vi "NodosPropiedad_Graficas.vi"() -> ()   [LabVIEW 2020]
uses:
  <vilib>/numeric/Random Number (Range) I64.vi
  <vilib>/numeric/sub_Random U32.vi
panel:
  out "Date and Time":string
  in  "Abort":bool
  in  "limite alto":dbl
  in  "Sample Rate (ms)":u32
  in  "Points to Acquired":i32
  out "Point Acquired":i32
  out "Fuera de rango":bool
  out "Temperatura":cluster{"number":i64, "limite alto":dbl}(graph)
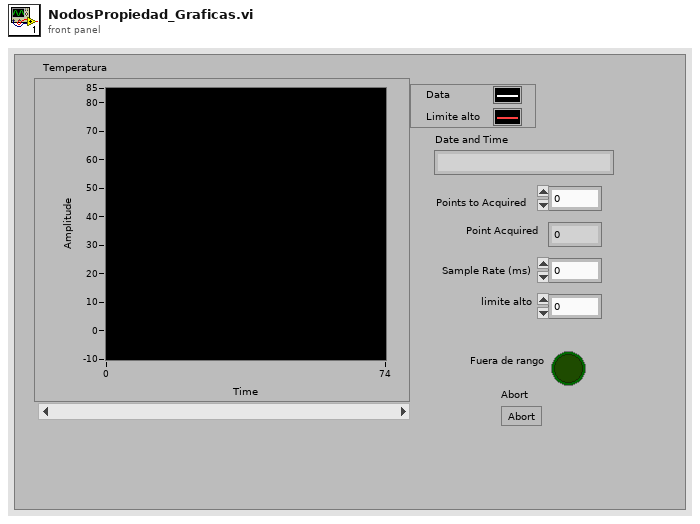
[diagram p1: front panel]
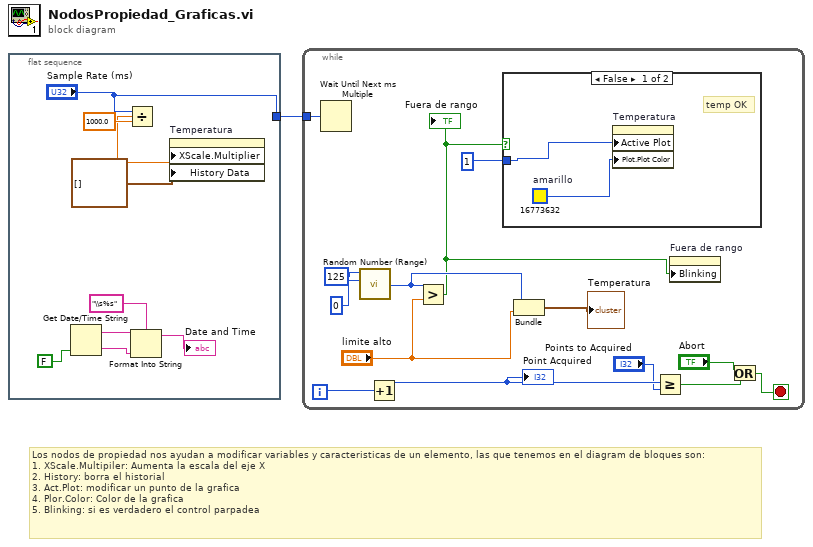
[diagram p0: block diagram]
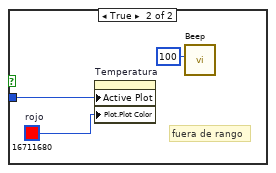
[diagram p2: hidden frame]
diagram:
  # "Los nodos de propiedad nos ayudan a modificar variables y caracteristicas de un elemento, las que tenemos en el diagram de bloques son:\n1. XScale.Multipiler: Aumenta la escala del eje X\n2. History: borra el historial  \n3. Act.Plot: modificar un punto de la grafica \n4. Plor.Color: Color de la grafica \n5. Blinking: si es verdadero el control parpadea"
  n1 = flat-sequence {
    tunnel: ["Sample Rate (ms)"] -> w1
    frame #0 {
      n2 = Get Date/Time String(want seconds? (F)=FALSE) -> (date string=w5:string, time string=w4:string)  [unwired: 2 in]
      n3 = Divide(x="Sample Rate (ms)", y=1000.0) -> (x/y=w9:dbl)
      n4 = Format Into String(format string="\\s%s", initial string=w5, w4) -> (resulting string=→"Date and Time":string)  [unwired: 1 in, 1 out]
      n5 = property on="Temperatura" class="WFChart (strict)"("XScale.Multiplier"=w9, "History Data"=cluster{"number":i64, "limite alto":dbl}[] []) -> ()  [unwired: 2 in, 2 out]
    }
  }
  n6 = while {
    tunnel: w1 -> [w11]
    i -> [w24]
    stop <- w23 stop-if-true
    n7 = Wait Until Next ms Multiple(millisecond multiple=w11) -> ()  [unwired: 1 out]
    n8 = call-poly <vilib>:"Random Number (Range).vi"("lower bound (-100)"=u64 0 ("lower bound (0)"), "upper bound (100)"=u64 125) -> ("number"=w18:i64)  [unwired: 9 in]
    n9 = Increment(x=w24) -> (x+1=w16:i32)
    "Point Acquired" <- w16
    n10 = Greater?(x=w18, y="limite alto") -> (0:w13:bool)
    "Fuera de rango" <- w13
    n11 = case shown="False" w13 {
      tunnel: u32 1 ("Active Plot") -> [w25 w29]
      frame False {
        w26 = u32 16773632  # amarillo
        # "temp OK"
        n12 = property on="Temperatura" class="WFChart (strict)"("Active Plot"=w25, "Plot.Plot Color"=w26) -> ()  [unwired: 2 in, 2 out]
      }
      frame True {
        w28 = u32 16711680  # rojo
        # "fuera de rango"
        n13 = property on="Temperatura" class="WFChart (strict)"("Active Plot"=w29, "Plot.Plot Color"=w28) -> ()  [unwired: 2 in, 2 out]
        n14 = call <vilib>:"Beep.vi"("duration (msec)"=u32 100) -> ()  [unwired: 11 in]
      }
    }
    n15 = Bundle("number"=w18, "limite alto"="limite alto") -> (→"Temperatura":cluster{"number":i64, "limite alto":dbl})  [unwired: 1 in]
    n16 = Greater Or Equal?(x=w16, y="Points to Acquired") -> (x >= y?=w22:bool)
    n17 = property on="Fuera de rango" class="Bool (strict)"("Blinking"=w13) -> ()  [unwired: 2 in, 2 out]
    n18 = Or(x="Abort", y=w22) -> (x .or. y?=w23:bool)
  }
